vi "ListThisLevelDependencies.vi"(8 "error in (no error)":errorcluster, 11 "SMO in":refnum<class "SMO.lvclass">) -> (0 "error out":errorcluster, 2 "[My Dependencies]":refnum<class "SMO.lvclass">[](array[class]), 3 "SMO out":refnum<class "SMO.lvclass">)   [LabVIEW 2019, in "SMO.lvclass"]
doc: "JKI State Machine Objects (SMO) 1.3.0.56\nJKI - JKI\nCopyright (c) 2017, JKI"
uses:
  SMO.lvclass
  <vilib>/regexp/Match Regular Expression.xnode
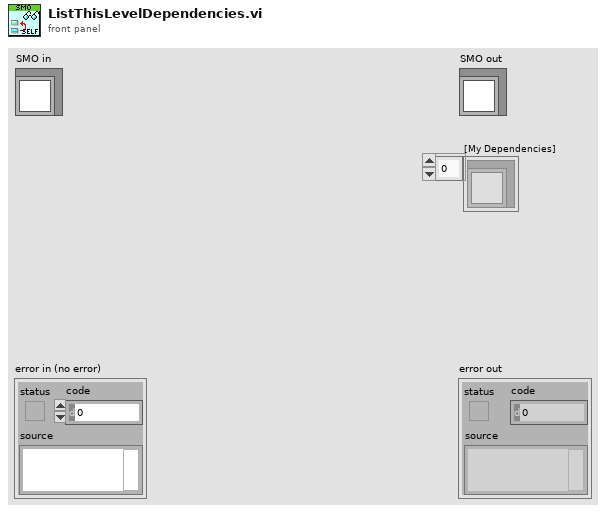
[diagram p1: front panel]
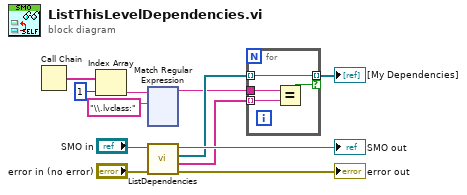
[diagram p0: block diagram]
diagram:
  n1 = Call Chain() -> (call chain=w5:string[])
  n2 = Index Array(array=w5, index=1) -> (element=w4:string)
  n3 = xnode "Match Regular Expression"("input string"=w4, "regular expression"="\\.lvclass:") -> ("before match"=w2:string)  [unwired: 4 in, 4 out]
  n4 = call "ListDependencies.vi"("error in (no error)"="error in (no error)", "SMO in"="SMO in") -> ("error out"=→"error out":errorcluster, "Level"=w6:string[], "[Dependencies]"=w7:refnum<class "SMO.lvclass">[], "SMO out"=→"SMO out":refnum<class "SMO.lvclass">)  [unwired: 6 in]
  n5 = for {
    tunnel: [w16] -> w12 mode=indexing if=w15
    tunnel: w7 -> [w16] mode=indexing
    tunnel: w6 -> [w14] mode=indexing
    tunnel: w2 -> [w13]
    n6 = Equal?(x=w13, y=w14) -> (x = y?=w15:bool)
  }
  "[My Dependencies]" <- w12
